vi "Read.vi"(8 "error in (no error)":errorcluster, 10 "# Channels (1)":i32=1, 11 "VISA Resource Name":refnum<visa-resource-name>) -> (0 "error out":errorcluster, 1 "# Readings":i32, 2 "Readings":string, 3 "VISA Resource Name Out":refnum<visa-resource-name>)   [LabVIEW 2012, in "Agilent 34970.lvlib"]
doc: "This VI allows you to read data from the instrument's output buffer. \n\nThe VI takes the maximum number of readings from the buffer such that there are an equal number of readings per channel. It returns the readings and the number of readings. You must wire the # Channels terminal.\n\nThis is an advanced measurment VI. For more information on the different ways to take and configure a measurment, refer to the context help and block diagram of \"HP34970A Advanced Scan Example.vi\"."
uses:
  <instrlib>/Agilent 34970/Agilent 34970.lvlib
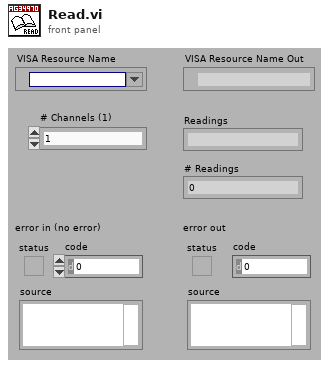
[diagram p1: front panel]
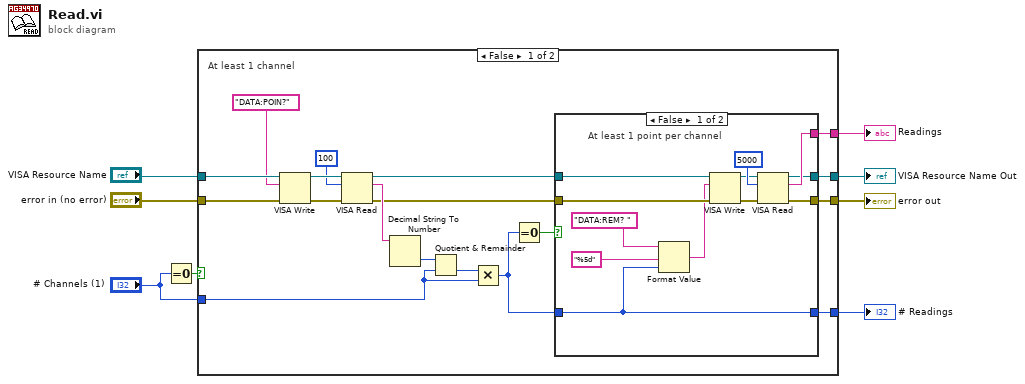
[diagram p0: block diagram]
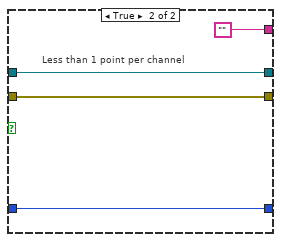
[diagram p2: hidden frame]
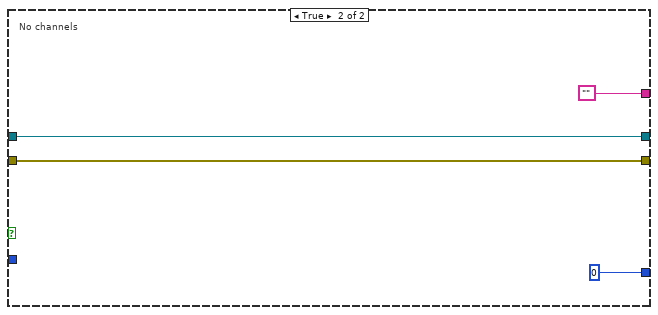
[diagram p3: hidden frame]
diagram:
  n1 = Equal To 0?(x="# Channels (1)") -> (x = 0?=w6:bool)
  n2 = case shown="False" w6 {
    tunnel: [w13 0] -> w7
    tunnel: [w10 ""] -> w8
    tunnel: "# Channels (1)" -> [w14 _]
    tunnel: [w12 w46] -> w4
    tunnel: [w11 w45] -> w3
    tunnel: "error in (no error)" -> [w15 w46]
    tunnel: "VISA Resource Name" -> [w16 w45]
    frame False {
      # "At least 1 channel"
      n3 = VISA Write(VISA resource name=w16, write buffer="DATA:POIN?", error in (no error)=w15) -> (VISA resource name out=w26:refnum<visa-resource-name>, error out=w25:errorcluster)  [unwired: 1 out]
      n4 = VISA Read(VISA resource name=w26, byte count=u32 100 ("byte count (0)"), error in (no error)=w25) -> (VISA resource name out=w22:refnum<visa-resource-name>, read buffer=w24:string, error out=w21:errorcluster)  [unwired: 1 out]
      n5 = Decimal String To Number(string=w24) -> (number=w18:i32)  [unwired: 2 in, 1 out]
      n6 = Quotient & Remainder(x=w18, y=w14) -> (floor(x/y)=w17:i32)  [unwired: 1 out]
      n7 = Multiply(x=w17, y=w14) -> (x*y=w19:i32)
      n8 = Equal To 0?(x=w19) -> (x = 0?=w20:bool)
      n9 = case shown="False" w20 {
        tunnel: w19 -> [w28 w39]
        tunnel: w21 -> [w38 w41]
        tunnel: w22 -> [w37 w42]
        tunnel: [w35 ""] -> w10
        tunnel: [w34 w41] -> w12
        tunnel: [w33 w42] -> w11
        tunnel: [w28 w39] -> w13
        frame False {
          # "At least 1 point per channel"
          n10 = Format Value(string ("")="DATA:REM? ", format string="%5d", value (0)=w28) -> (output string=w27:string)
          n11 = VISA Write(VISA resource name=w37, write buffer=w27, error in (no error)=w38) -> (VISA resource name out=w30:refnum<visa-resource-name>, error out=w31:errorcluster)  [unwired: 1 out]
          n12 = VISA Read(VISA resource name=w30, byte count=u32 5000 ("byte count (0)"), error in (no error)=w31) -> (VISA resource name out=w33:refnum<visa-resource-name>, read buffer=w35:string, error out=w34:errorcluster)  [unwired: 1 out]
        }
        frame True {
          # "Less than 1 point per channel"
        }
      }
    }
    frame True {
      # "No channels"
    }
  }
  "Readings" <- w8
  "# Readings" <- w7
  "error out" <- w4
  "VISA Resource Name Out" <- w3
